vi "RegisterMap_ScanFile.vi"(8 "error in (no error)":errorcluster, 11 "Register Map File":path) -> (0 "error out":errorcluster, 1 "Register Names":string[](array[string]), 2 "Register RegMap Data":string[](array[string]), 3 "ADC Registers":T1[](array[typedef]) {"Base" format="%.0x"; "Item Count" format="%.0x"; "Value" format="%.0x"; "RegMap"."Mask" format="%.0x"; "Default" format="%.0x"; "Register" format="%.0x"})   [LabVIEW 2010]
doc: "This VI scans in the regsiter map data from a text file.\n(see block diagram for text file format)\n\nInputs:\nRegister Map File - (path) path and filename of the register map text file\nerror in - error input cluster\n\nOutputs:\nAMC7812 Registers - (cluster[]) array of clusters containing the regsiter map data\nRegsiter Names - (str[]) array of strings containing the register names; to be used for searching\nRegister RegMap Data - (str[]) array of string containing the \"Register String\" information to be parsed and sorted.\nerror out - error output cluster"
uses:
  TYP_ADSxxxx Register.ctl
  TYP_RegMap Item.ctl
  <vilib>/Utility/file.llb/Read From Spreadsheet File (string).vi
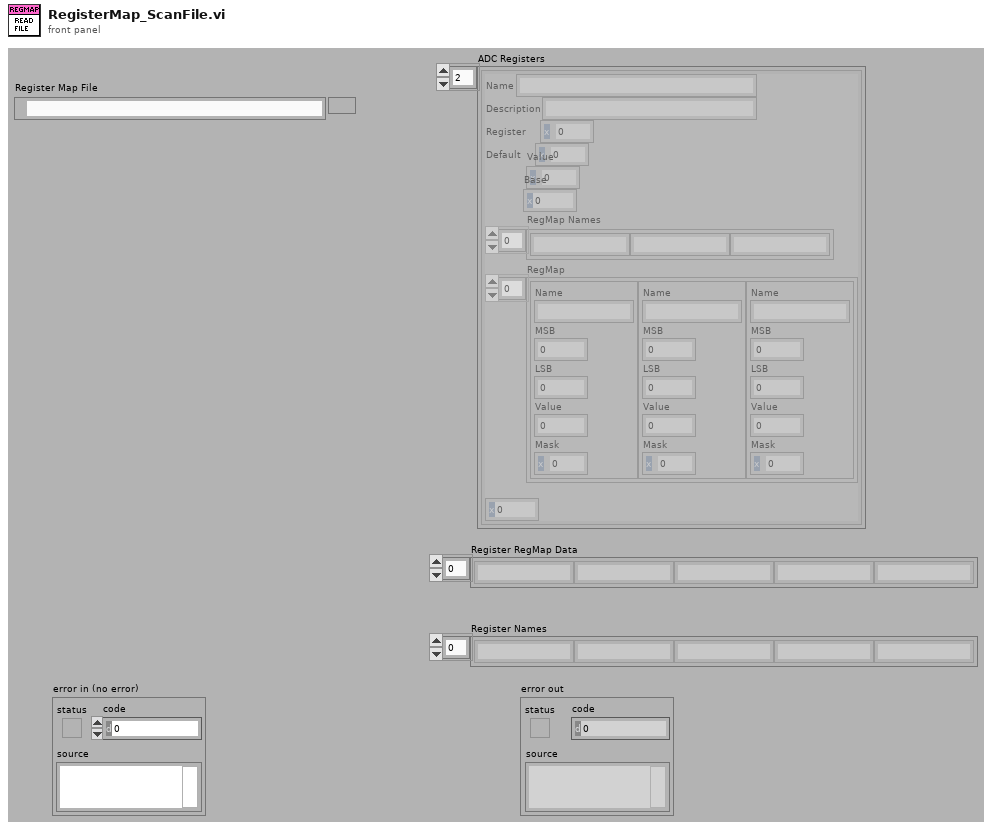
[diagram p1: front panel]
types:
  T1 = typedef "TYP_ADSxxxx Register.ctl" = cluster{"Name":string, "Description":string, "Register":u16, "Default":u16, "Value":u16, "Base":u16, "RegMap Names":string[], "RegMap":T2[], "Item Count":u8}
  T2 = typedef "TYP_RegMap Item.ctl" = cluster{"Name":string, "MSB":u16, "LSB":u16, "Value":u16, "Mask":u16}
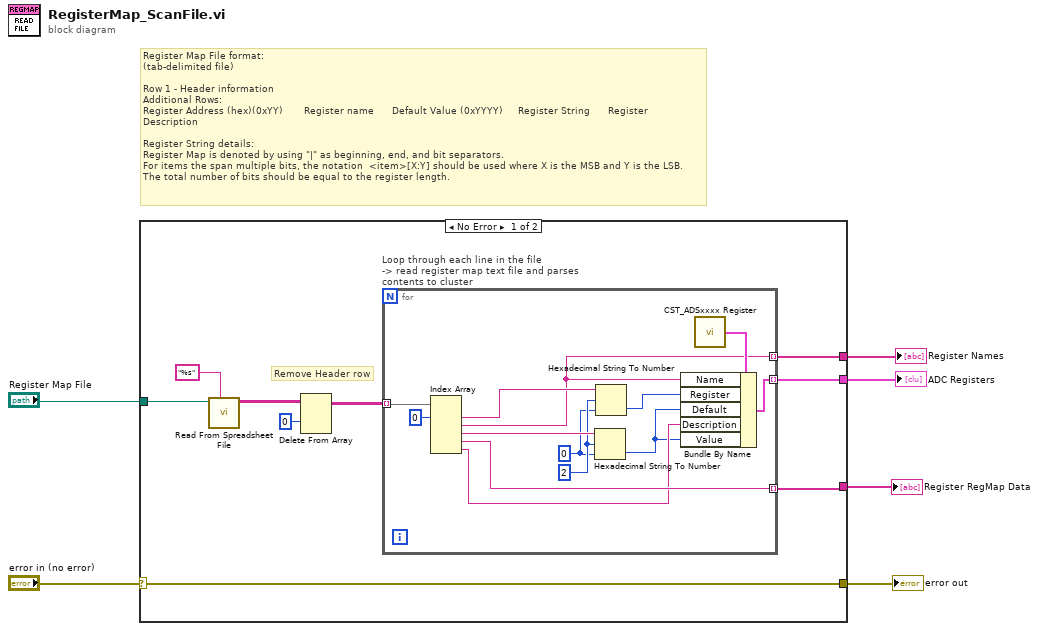
[diagram p0: block diagram]
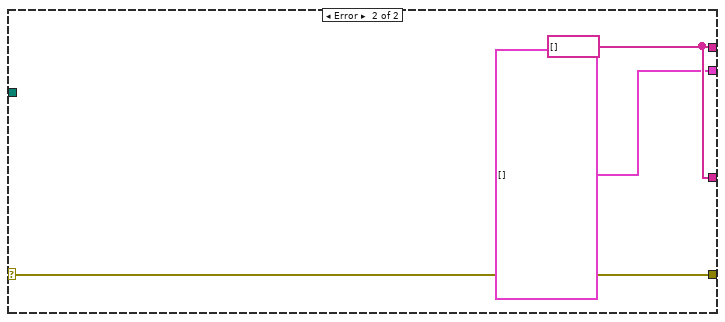
[diagram p2: hidden frame]
diagram:
  # "Register Map File format:\n(tab-delimited file)\n\nRow 1 - Header information\nAdditional Rows:\nRegister Address (hex)(0xYY)       Register name      Default Value (0xYYYY)     Register String      Register Description\n\nRegister String details:\nRegister Map is denoted by using \"|\" as beginning, end, and bit separators.  \nFor items the span multiple bits, the notation  <item>[X:Y] should be used where X is the MSB and Y is the LSB.\nThe total number of bits should be equal to the register length."
  n1 = case shown="No Error" "error in (no error)" {
    selector: "error in (no error)" -> [w10 w31]
    tunnel: "Register Map File" -> [w14 _]
    tunnel: [w10 w31] -> w4
    tunnel: [w8 w30] -> w3
    tunnel: [w9 w30] -> w2
    tunnel: [w7 T1[] []] -> w1
    frame No Error {
      # "Remove Header row"
      n2 = call-poly <vilib>:"Read From Spreadsheet File.vi"("format (%s)"="%s" ("format (%.3f)"), "file path (dialog if empty)"=w14) -> ("all rows"=w13:string[][])  [unwired: 2 in, 7 out]
      n3 = Delete From Array(array=w13, index (row)=0) -> (array with subset deleted=w11:string[][])  [unwired: 2 in, 1 out]
      n4 = for "Loop through each line in the file\n-> read register map text file and parses contents to cluster" {
        tunnel: w11 -> [w28] mode=indexing
        tunnel: [w24] -> w9 mode=indexing
        tunnel: [w20] -> w8 mode=indexing
        tunnel: [w19] -> w7 mode=indexing
        w22 = u32 0 ("offset")
        w23 = 2 ("offset")
        n5 = Index Array(array=w28, index #1=0 ("index")) -> (element #1=w27:string, element #2=w20:string, element #3=w25:string, element #4=w24:string, element #5=w17:string)  [unwired: 4 in]
        n6 = Hexadecimal String To Number(string=w25, offset=w23, default (0uL)=w22) -> (number=w16:u32)  [unwired: 1 out]
        n7 = Hexadecimal String To Number(string=w27, offset=w23, default (0uL)=w22) -> (number=w18:u32)  [unwired: 1 out]
        n8 = call "CST_ADSxxxx Register.vi"() -> ("ADC Register"=w21:T1)  [unwired: 1 out]
        n9 = Bundle By Name(cluster=w21, "Name"=w20, "Register"=w18, "Default"=w16, "Description"=w17, "Value"=w16) -> (w19:T1)
      }
    }
    frame Error {
      w30 = string[] []
    }
  }
  "error out" <- w4
  "Register Names" <- w3
  "Register RegMap Data" <- w2
  "ADC Registers" <- w1
